vi "QO_Error_Logger.vi"(0 "Queue_Name_In":string, 1 "Max_Queue_Size_In":i32=-1, 5 "Time_Out_In_ms (-1)":i32=10, 7 "Data_In":T1, 11 "Error_In":errorcluster, 13 "Queue_Operation":T5=enum."Flush") -> (3 "Max_Queue_Size_Out":i32=-1, 4 "Queue_Name_Out":string, 6 "timed out?":bool, 8 "Data_Out":T1, 15 "Error_Out":errorcluster)   [LabVIEW 2021]
doc: "Used to transfer data from one vi to another using queue."
uses:
  Controls/Queue_Operation.ctl
  Controls/Logger_Data.ctl
  Controls/Generated_data.ctl
  Controls/Current_Limit.ctl
  Controls/Temperature_Limit.ctl
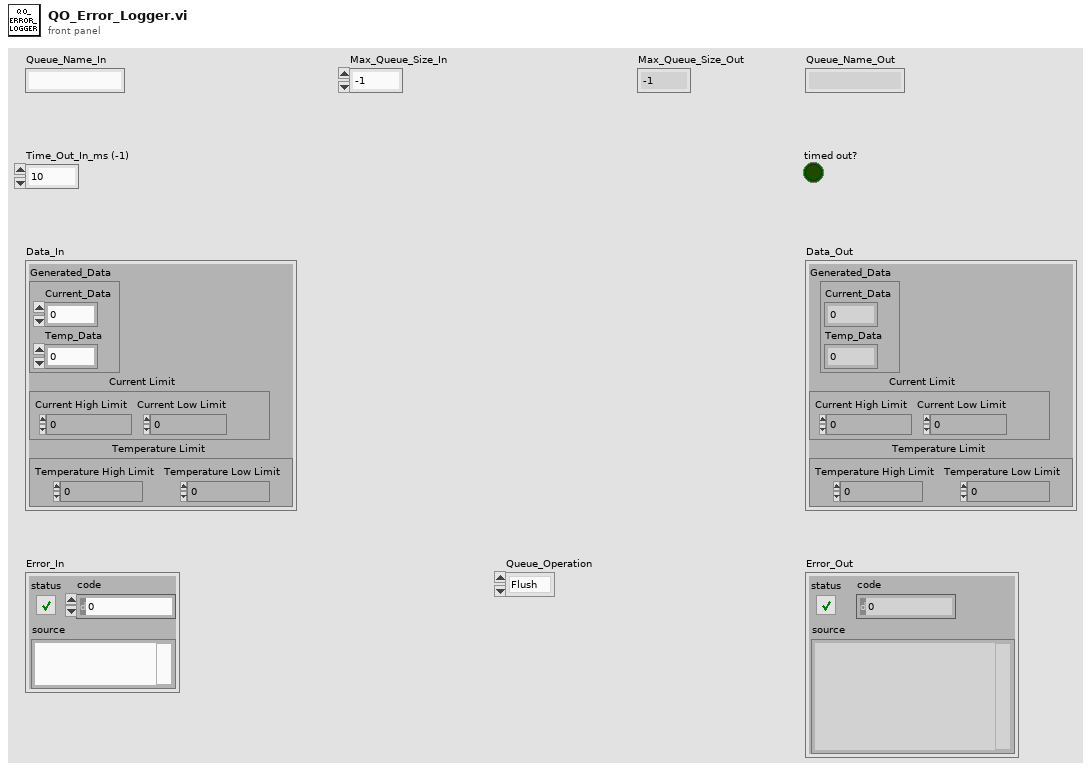
[diagram p1: front panel]
types:
  T1 = typedef "Logger_Data.ctl" = cluster{"Generated_Data":T2, "Current_Limit":T3, "Temperature_Limit":T4}
  T2 = typedef "Generated_data.ctl" = cluster{"Current_Data":dbl, "Temp_Data":dbl}
  T3 = typedef "Current_Limit.ctl" = cluster{"Current_High_Limit":dbl, "Current_Low_Limit":dbl}
  T4 = typedef "Temperature_Limit.ctl" = cluster{"Temperature_High_Limit":dbl, "Temperature_Low_Limit":dbl}
  T5 = typedef "Queue_Operation.ctl" = enum16{"Obtain_Queue", "Enqueue", "Lossy_Enqueue", "Preview", "Queue_Status", "Release_Queue", "Dequeue", "Flush"}
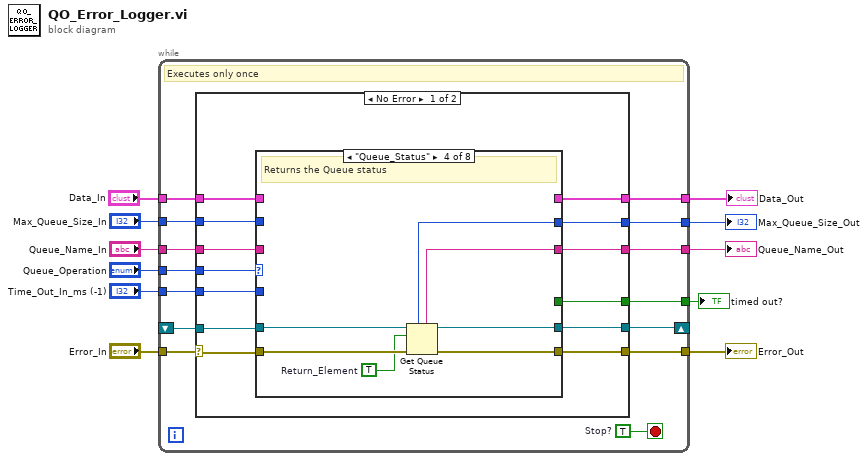
[diagram p0: block diagram]
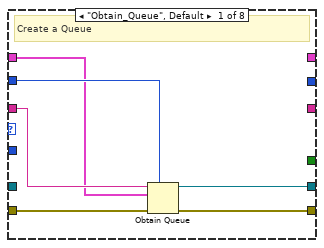
[diagram p2: hidden frame]
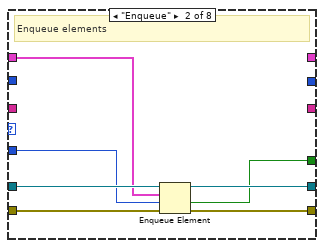
[diagram p3: hidden frame]
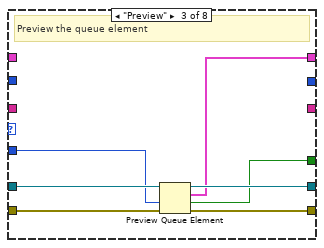
[diagram p4: hidden frame]
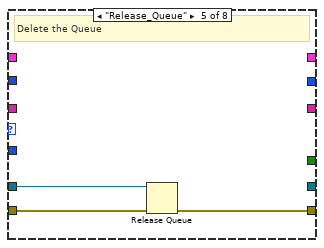
[diagram p5: hidden frame]
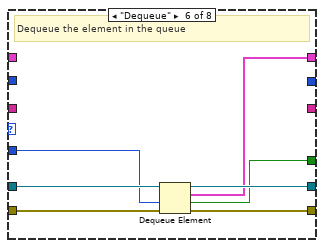
[diagram p6: hidden frame]
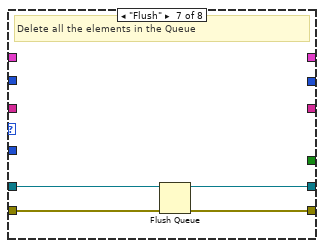
[diagram p7: hidden frame]
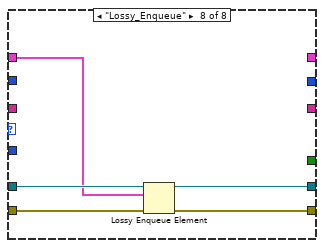
[diagram p8: hidden frame]
diagram:
  n1 = while {
    tunnel: "Max_Queue_Size_In" -> [w25]
    tunnel: "Time_Out_In_ms (-1)" -> [w22]
    tunnel: [w20] -> w8
    tunnel: "Queue_Operation" -> [w17]
    shift-right: [w18] -> _
    shift-left: _ -> [w14]
    tunnel: "Data_In" -> [w23]
    tunnel: [w21] -> w2
    tunnel: "Queue_Name_In" -> [w16]
    tunnel: [w19] -> w7
    tunnel: "Error_In" -> [w15]
    tunnel: [w24] -> w10
    tunnel: [w12] -> w1
    stop <- w13 stop-if-true
    w13 = TRUE  # Stop?
    # "Executes only once"
    n2 = case shown="No Error" w15 {
      selector: w15 -> [w28 w86]
      tunnel: w17 -> [w29 _]
      tunnel: w16 -> [w30 _]
      tunnel: w25 -> [w38 _]
      tunnel: [w37 w85] -> w18
      tunnel: [w36 w86] -> w24
      tunnel: w23 -> [w31 _]
      tunnel: w22 -> [w35 _]
      tunnel: [w34 _] -> w21
      tunnel: [w33 _] -> w20
      tunnel: [w32 _] -> w19
      tunnel: w14 -> [w27 w85]
      tunnel: [w26 _] -> w12
      frame No Error {
        n3 = case shown="\"Queue_Status\"" w29 {
          tunnel: w28 -> [w44 w51 w57 w64 w68 w74 w78 w83]
          tunnel: w30 -> [w42 _ _ _ _ _ _ _]
          tunnel: w38 -> [w41 _ _ _ _ _ _ _]
          tunnel: [w39 w47 w56 w63 _ w73 w77 w82] -> w37
          tunnel: [w43 w50 w55 w62 w67 w71 w76 w81] -> w36
          tunnel: w27 -> [_ w49 w58 w65 w66 w75 w79 w84]
          tunnel: w31 -> [w40 w48 _ _ _ _ _ w80]
          tunnel: w35 -> [_ w46 w54 _ _ w70 _ _]
          tunnel: [_ _ w53 _ _ w72 _ _] -> w34
          tunnel: [_ _ _ w61 _ _ _ _] -> w33
          tunnel: [_ _ _ w60 _ _ _ _] -> w32
          tunnel: [_ w45 w52 _ _ w69 _ _] -> w26
          frame "Obtain_Queue", Default {
            # "Create a Queue"
            n4 = Obtain Queue(max queue size (-1, unlimited)=w41, name (unnamed)=w42, element data type=w40, error in (no error)=w44) -> (queue out=w39:refnum<queue>, error out=w43:errorcluster)  [unwired: 1 in, 1 out]
          }
          frame "Enqueue" {
            # "Enqueue elements"
            n5 = Enqueue Element(queue=w49, element=w48, timeout in ms (-1)=w46, error in (no error)=w51) -> (queue out=w47:refnum<queue>, timed out?=w45:bool, error out=w50:errorcluster)
          }
          frame "Preview" {
            # "Preview the queue element"
            n6 = Preview Queue Element(queue=w58, timeout in ms (-1)=w54, error in (no error)=w57) -> (queue out=w56:refnum<queue>, element=w53:T1, timed out?=w52:bool, error out=w55:errorcluster)
          }
          frame "Queue_Status" {
            w59 = TRUE  # Return_Element
            # "Returns the Queue status"
            n7 = Get Queue Status(queue=w65, return elements? (F)=w59, error in (no error)=w64) -> (queue out=w63:refnum<queue>, queue name=w60:string, max queue size=w61:i32, error out=w62:errorcluster)  [unwired: 4 out]
          }
          frame "Release_Queue" {
            # "Delete the Queue"
            n8 = Release Queue(queue=w66, error in (no error)=w68) -> (error out=w67:errorcluster)  [unwired: 1 in, 2 out]
          }
          frame "Dequeue" {
            # "Dequeue the element in the queue"
            n9 = Dequeue Element(queue=w75, timeout in ms (-1)=w70, error in (no error)=w74) -> (queue out=w73:refnum<queue>, element=w72:T1, timed out?=w69:bool, error out=w71:errorcluster)
          }
          frame "Flush" {
            # "Delete all the elements in the Queue"
            n10 = Flush Queue(queue=w79, error in (no error)=w78) -> (queue out=w77:refnum<queue>, error out=w76:errorcluster)  [unwired: 1 out]
          }
          frame "Lossy_Enqueue" {
            n11 = Lossy Enqueue Element(queue=w84, element=w80, error in (no error)=w83) -> (queue out=w82:refnum<queue>, error out=w81:errorcluster)  [unwired: 2 out]
          }
        }
      }
      frame Error {
      }
    }
  }
  "Error_Out" <- w10
  "Max_Queue_Size_Out" <- w8
  "Queue_Name_Out" <- w7
  "Data_Out" <- w2
  "timed out?" <- w1
